vi "Qrcode Exercise Array Timeout Scan Run.vi"() -> ()   [LabVIEW 2019]
uses:
  <vilib>/userDefined/High Color/IMAQdx.ctl
  <vilib>/vision/driver/NI_Vision_Acquisition_Software.lvlib
  <vilib>/vision/NI_Vision_Development_Module.lvlib
panel:
  out "Base 3 El 3":string
  out "Base 3 El 2":string
  out "Base 3 El 1":string
  out "Base 2 El 3":string
  out "Base 2 El 2":string
  out "Base 2 El 1":string
  out "Base 1 El 3":string
  out "Base 1 El 2":string
  out "Base 1 El 1":string
  out "Base 3":string[](array[string])
  out "Base 2":string[](array[string])
  out "Base 1":string[](array[string])
  out "Index ke":i32
  out "Found?":bool
  out "Data":string
  out "Image":T1(plugin-control)
  out "Code":string
  out "Option 2":enum16{"scan", "run", "timeout"}(ring)
  out "Option":enum16{"qrcode", "lampu"}(ring)
  out "Blue":bool
  out "Green":bool
  out "Yellow":bool
  in  "Main":T2(array[cluster])=[{"Option"=enum."qrcode", "Option 2"=enum."scan", "Code"=""}, {"Option"=enum."qrcode", "Option 2"=enum."scan", "Code"=""}, {"Option"=enum."qrcode", "Option 2"=enum."scan", "Code"=""}, {"Option"=enum."qrcode", "Option 2"=enum."run", "Code"=""}, {"Option"=enum."qrcode", "Option 2"=enum."run", "Code"=""}, {"Option"=enum."qrcode", "Option 2"=enum."run", "Code"=""}, {"Option"=enum."lampu", "Option 2"=enum."timeout", "Code"=""}, {"Option"=enum."lampu", "Option 2"=enum."timeout", "Code"=""}, {"Option"=enum."lampu", "Option 2"=enum."timeout", "Code"=""}]
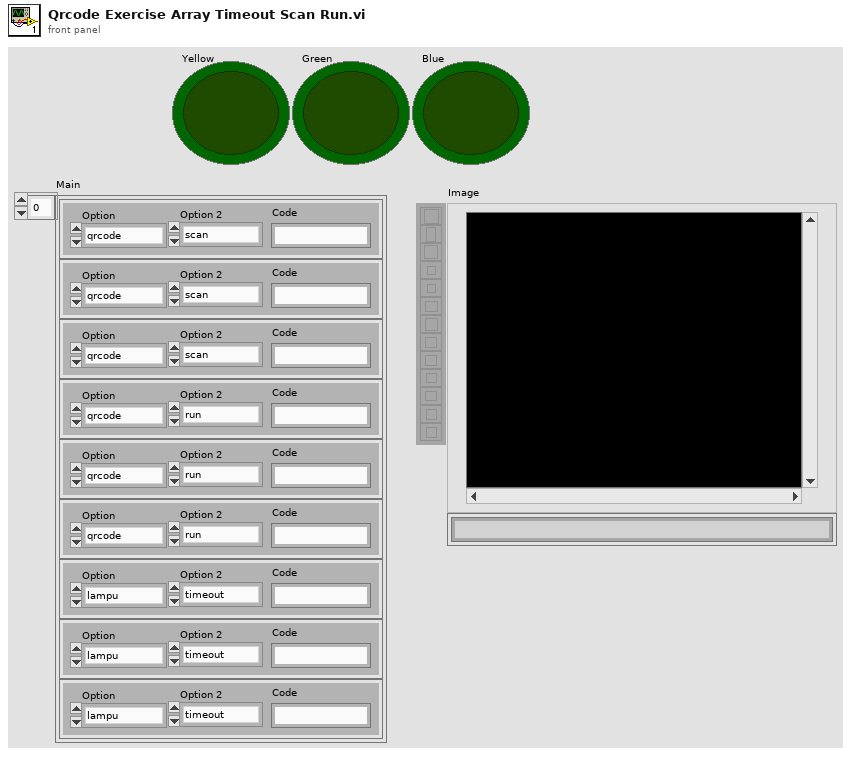
[diagram p1: front panel]
types:
  T1 = typedef "IMAQ Image.ctl" = refnum<image>
  T2 = cluster{"Option":enum16{"qrcode", "lampu"}, "Option 2":enum16{"scan", "run", "timeout"}, "Code":string}[]
  T3 = cluster{"Option":enum16{"qrcode", "lampu"}, "Option 2":enum16{"scan", "run", "timeout"}, "Code":string}
  T4 = typedef "IMAQdx.ctl" = refnum<k21>
  T5 = typedef "Image Type" = u32
  T6 = typedef "QR Code Report.ctl" = cluster{"Found?":bool, "Data":string, "Bounding Box":cluster{"x":sgl, "y":sgl}[], "Errors Corrected":u32, "Dimensions (Rows/Cols)":u32, "Version":u32, "QR Model":T7, "Stream Mode":T8, "Barcode Polarity":T9, "Mirrored?":bool, "Append Stream Position":u32, "Size of Append Stream":u32, "First EAN-128 ID":i32, "First Alternate Language ID":i32, "Append Stream ID":u32, "Minimum Edge Strength":u32, "Demodulation Mode":T10, "Cell Sample Size":T11, "Cell Filter Mode":T12}
  T7 = typedef "QR Code Model Type.ctl" = i32
  T8 = typedef "QR Code Stream Mode Type.ctl" = i32
  T9 = typedef "Data Matrix Polarity.ctl" = i32
  T10 = typedef "Demodulation Mode.ctl" = i32
  T11 = typedef "Cell Sample Size.ctl" = i32
  T12 = typedef "Cell Filter Mode.ctl" = i32
  T13 = cluster{"Option":enum16{"qrcode", "lampu"}, "Option 2":enum16{"scan", "run", "timeout"}, "Data":string}
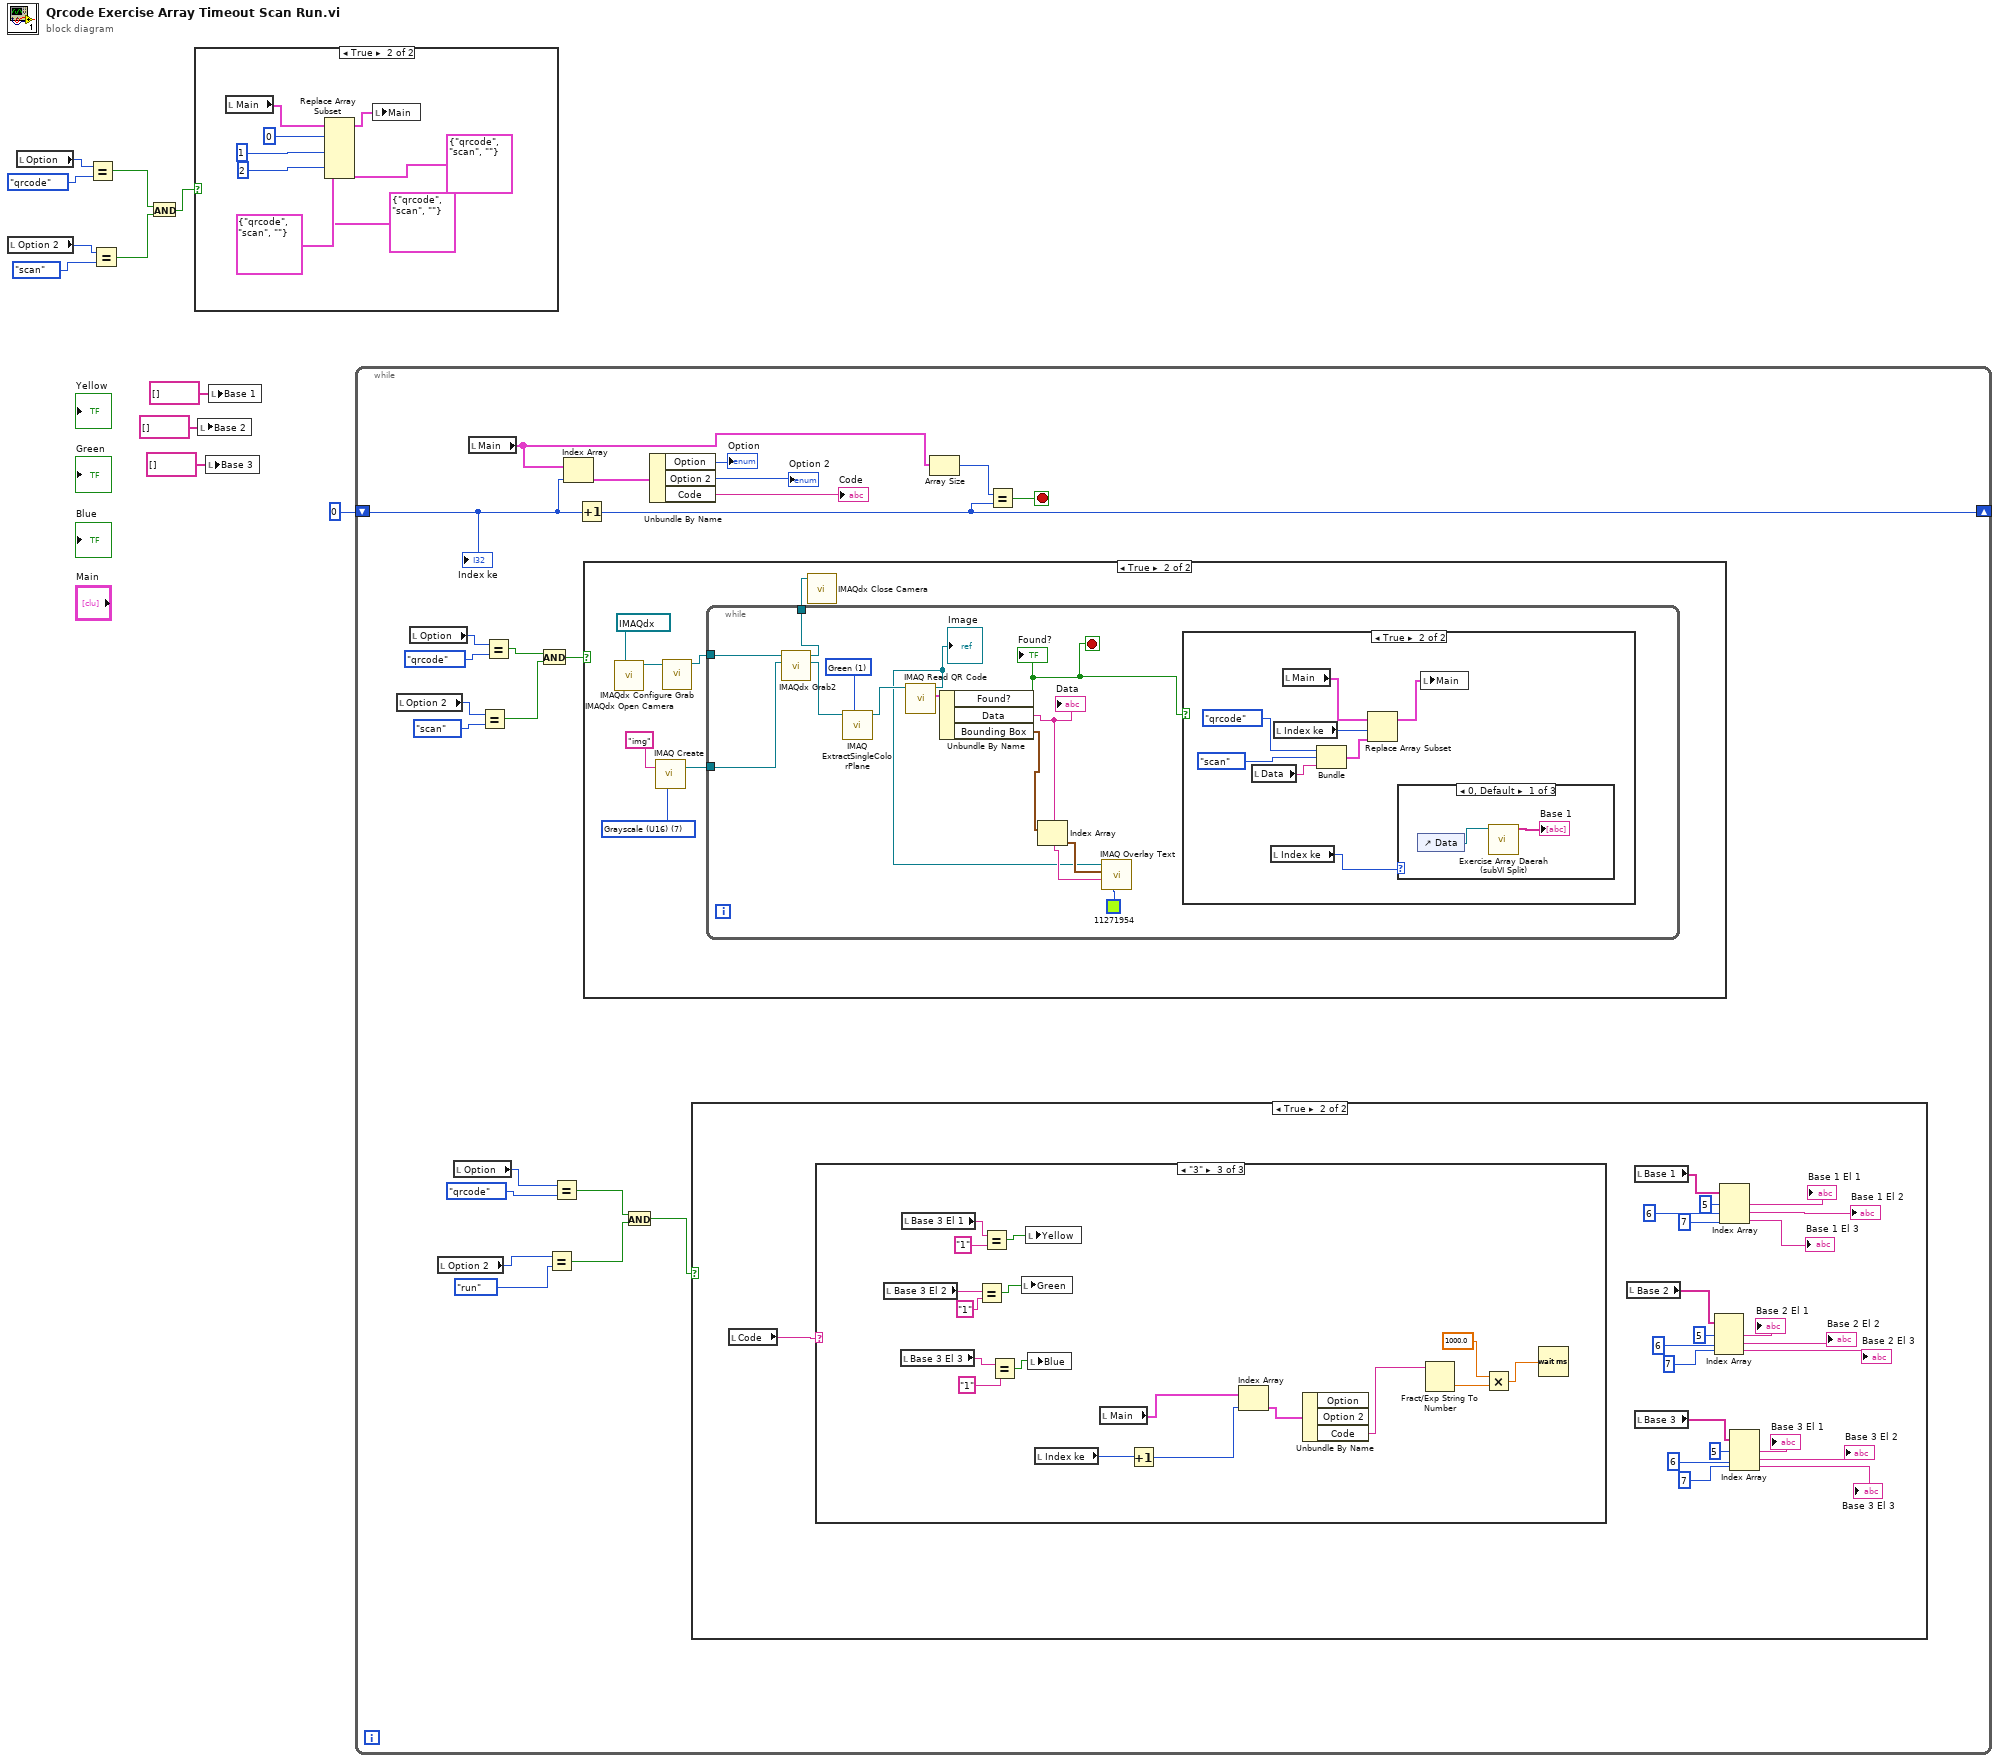
[diagram p0: block diagram]
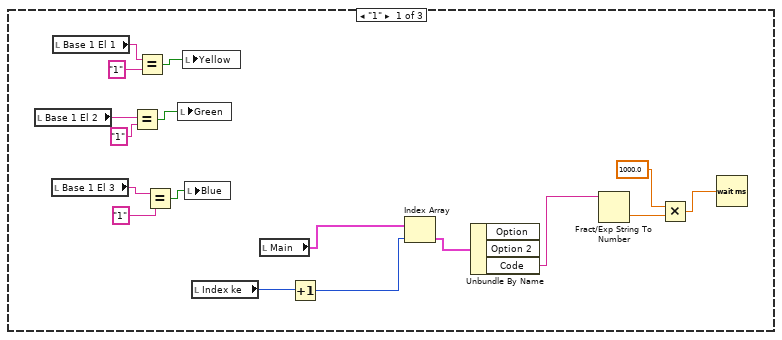
[diagram p4: hidden frame]
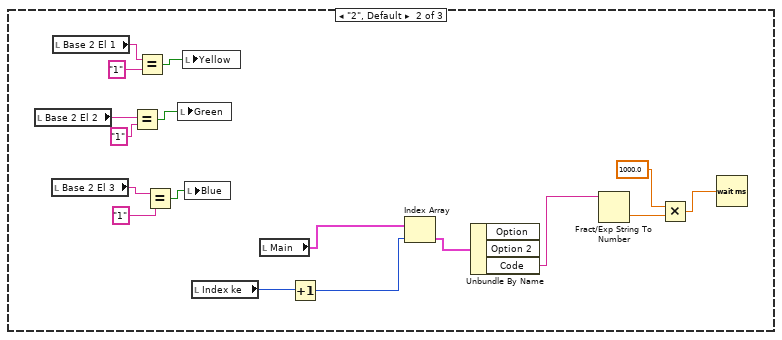
[diagram p5: hidden frame]
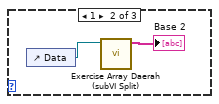
[diagram p8: hidden frame]
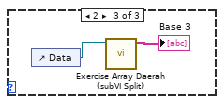
[diagram p9: hidden frame]
diagram:
  n1 = local read "Option 2"() -> (w10:enum16{"scan", "run", "timeout"})
  n2 = local read "Option"() -> (w8:enum16{"qrcode", "lampu"})
  n3 = Equal?(x=w8, y=enum16{"qrcode", "lampu"}."qrcode" ("Option")) -> (x = y?=w6:bool)
  n4 = Equal?(x=w10, y=enum16{"scan", "run", "timeout"}."scan" ("Option 2")) -> (x = y?=w5:bool)
  n5 = And(x=w6, y=w5) -> (x .and. y?=w4:bool)
  n6 = case shown="True" w4 {
    frame False {
    }
    frame True {
      n7 = local read "Main"() -> (w19:T2)
      n8 = Replace Array Subset(array=w19, new element #1=T3 {"Option"=enum."qrcode", "Option 2"=enum."scan", "Code"=""} ("new element/subarray"), index #1=0 ("index"), new element #2=T3 {"Option"=enum."qrcode", "Option 2"=enum."scan", "Code"=""} ("new element/subarray"), index #2=1 ("index"), new element #3=T3 {"Option"=enum."qrcode", "Option 2"=enum."scan", "Code"=""} ("new element/subarray"), index #3=2 ("index")) -> (w12:T2)
      n9 = local write "Main"(w12) -> ()
    }
  }
  n10 = local write "Base 2"(string[] [] ("Base 2")) -> ()
  n11 = local write "Base 3"(string[] [] ("Base 3")) -> ()
  n12 = local write "Base 1"(string[] [] ("Base 1")) -> ()
  n13 = while {
    shift-right: [w35] -> _
    shift-left: 0 -> [w42]
    stop <- w34 stop-if-true
    n14 = local read "Option 2"() -> (w32:enum16{"scan", "run", "timeout"})
    n15 = local read "Option"() -> (w31:enum16{"qrcode", "lampu"})
    n16 = local read "Option 2"() -> (w24:enum16{"scan", "run", "timeout"})
    n17 = local read "Option"() -> (w26:enum16{"qrcode", "lampu"})
    n18 = local read "Main"() -> (w37:T2)
    n19 = Equal?(x=w32, y=enum16{"scan", "run", "timeout"}."scan" ("Option 2")) -> (x = y?=w28:bool)
    n20 = Equal?(x=w31, y=enum16{"qrcode", "lampu"}."qrcode" ("Option")) -> (x = y?=w29:bool)
    n21 = And(x=w29, y=w28) -> (x .and. y?=w27:bool)
    n22 = Equal?(x=w24, y=enum16{"scan", "run", "timeout"}."run" ("Option 2")) -> (x = y?=w22:bool)
    n23 = Equal?(x=w26, y=enum16{"qrcode", "lampu"}."qrcode" ("Option")) -> (x = y?=w21:bool)
    n24 = Index Array(array=w37, index=w42) -> (element=w41:T3)
    n25 = Increment(x=w42) -> (x+1=w35:i32)
    n26 = case shown="True" w27 {
      frame False {
      }
      frame True {
        w120 = T5 7 items=["Grayscale (U8)", "Grayscale (I16)", "Grayscale (SGL)", "Complex (CSG)", "RGB (U32)", "HSL (U32)", "RGB (U64)", "Grayscale (U16)"] ("Image Type")
        n27 = call <vilib>:"IMAQdx Open Camera.vi"("Session In"=T4 "cam0") -> ("Session Out"=w122:T4)  [unwired: 9 in, 1 out]
        n28 = call "IMAQ Create"("Image Name"="img", "Image Type"=w120) -> ("New Image"=w116:T1)  [unwired: 3 in, 1 out]
        n29 = call <vilib>:"IMAQdx Configure Grab.vi"("Session In"=w122) -> ("Session Out"=w118:T4)  [unwired: 9 in, 1 out]
        n30 = while {
          tunnel: w118 -> [w135]
          tunnel: [w134] -> w117
          tunnel: w116 -> [w129]
          stop <- w123 stop-if-true
          w132 = 1 items=["Red", "Green", "Blue", "Hue", "Saturation", "Luminance", "Value", "Intensity"] ("Color Plane")
          n31 = call <vilib>:"IMAQdx Grab2.vi"("Image In"=w129, "Session In"=w135) -> ("Image Out"=w133:T1, "Session Out"=w134:T4)  [unwired: 6 in, 2 out]
          n32 = call "IMAQ ExtractSingleColorPlane"("Color Plane"=w132, "Image Src"=w133) -> ("Image Dst Out"=w131:T1)  [unwired: 8 in, 1 out]
          n33 = call "IMAQ Read QR Code"("Image"=w131) -> ("QR Code Report"=w130:T6, "Image (duplicate)"=w124:T1)  [unwired: 7 in, 2 out]
          "Image" <- w124
          n34 = Unbundle By Name(w130) -> ("Found?"=w123:bool, "Data"=w125:string, "Bounding Box"=w127:cluster{"x":sgl, "y":sgl}[])
          "Data" <- w125
          "Found?" <- w123
          n35 = Index Array(array=w127) -> (element=w126:cluster{"x":sgl, "y":sgl})  [unwired: 1 in]
          n36 = call "IMAQ Overlay Text"("Text Color (black)"=u32 11271954, "String"=w125, "Origin"=w126, "Image"=w124) -> ()  [unwired: 6 in, 2 out]
          n37 = case shown="True" w123 {
            frame False {
            }
            frame True {
              n38 = local read "Data"() -> (w139:string)
              n39 = local read "Index ke"() -> (w136:i32)
              n40 = local read "Index ke"() -> (w137:i32)
              n41 = local read "Main"() -> (w138:T2)
              n42 = Bundle("Option"=enum16{"qrcode", "lampu"}."qrcode", "Option 2"=enum16{"scan", "run", "timeout"}."scan", "Data"=w139) -> (w141:T13)  [unwired: 1 in]
              n43 = Replace Array Subset(array=w138, new element=w141, index=w137) -> (w140:T2)
              n44 = case shown="0, Default" w136 {
                frame 0, Default {
                  n45 = control-ref of="Data"() -> (w144:refnum<vi>)
                  n46 = call "Exercise Array Daerah (subVI Split).vi"("String in"=w144) -> ("Array"=→"Base 1":string[])  [unwired: 10 in]
                }
                frame 1 {
                  n47 = control-ref of="Data"() -> (w146:refnum<vi>)
                  n48 = call "Exercise Array Daerah (subVI Split).vi"("String in"=w146) -> ("Array"=→"Base 2":string[])  [unwired: 10 in]
                }
                frame 2 {
                  n49 = control-ref of="Data"() -> (w148:refnum<vi>)
                  n50 = call "Exercise Array Daerah (subVI Split).vi"("String in"=w148) -> ("Array"=→"Base 3":string[])  [unwired: 10 in]
                }
              }
              n51 = local write "Main"(w140) -> ()
            }
          }
        }
        n52 = call <vilib>:"IMAQdx Close Camera.vi"("Session In"=w117) -> ()  [unwired: 10 in, 1 out]
      }
    }
    n53 = And(x=w21, y=w22) -> (x .and. y?=w20:bool)
    n54 = Unbundle By Name(w41) -> ("Option"=→"Option":enum16{"qrcode", "lampu"}, "Option 2"=→"Option 2":enum16{"scan", "run", "timeout"}, "Code"=→"Code":string)
    n55 = case shown="True" w20 {
      frame False {
      }
      frame True {
        n56 = local read "Code"() -> (w64:string)
        n57 = case shown="\"3\"" w64 {
          frame "1" {
            n58 = local read "Base 1 El 2"() -> (w79:string)
            n59 = local read "Base 1 El 3"() -> (w80:string)
            n60 = local read "Base 1 El 1"() -> (w78:string)
            n61 = Equal?(x=w79, y="1") -> (x = y?=w73:bool)
            n62 = Equal?(x=w78, y="1") -> (x = y?=w81:bool)
            n63 = Equal?(x=w80, y="1") -> (x = y?=w74:bool)
            n64 = local write "Green"(w73) -> ()
            n65 = local write "Yellow"(w81) -> ()
            n66 = local write "Blue"(w74) -> ()
            n67 = local read "Index ke"() -> (w71:i32)
            n68 = local read "Main"() -> (w72:T2)
            n69 = Increment(x=w71) -> (x+1=w70:i32)
            n70 = Index Array(array=w72, index=w70) -> (element=w69:T3)
            n71 = Unbundle By Name(w69) -> ("Code"=w68:string)  [unwired: 2 out]
            n72 = Fract/Exp String To Number(string=w68) -> (number=w67:dbl)  [unwired: 3 in, 1 out]
            n73 = Multiply(x=1000.0, y=w67) -> (x*y=w65:dbl)
            n74 = Wait (ms)(milliseconds to wait=w65) -> ()  [unwired: 1 out]
          }
          frame "2", Default {
            n75 = local read "Base 2 El 2"() -> (w96:string)
            n76 = local read "Base 2 El 3"() -> (w97:string)
            n77 = local read "Base 2 El 1"() -> (w95:string)
            n78 = Equal?(x=w96, y="1") -> (x = y?=w90:bool)
            n79 = Equal?(x=w95, y="1") -> (x = y?=w98:bool)
            n80 = Equal?(x=w97, y="1") -> (x = y?=w91:bool)
            n81 = local write "Green"(w90) -> ()
            n82 = local write "Yellow"(w98) -> ()
            n83 = local write "Blue"(w91) -> ()
            n84 = local read "Index ke"() -> (w88:i32)
            n85 = local read "Main"() -> (w89:T2)
            n86 = Increment(x=w88) -> (x+1=w87:i32)
            n87 = Index Array(array=w89, index=w87) -> (element=w86:T3)
            n88 = Unbundle By Name(w86) -> ("Code"=w85:string)  [unwired: 2 out]
            n89 = Fract/Exp String To Number(string=w85) -> (number=w84:dbl)  [unwired: 3 in, 1 out]
            n90 = Multiply(x=1000.0, y=w84) -> (x*y=w82:dbl)
            n91 = Wait (ms)(milliseconds to wait=w82) -> ()  [unwired: 1 out]
          }
          frame "3" {
            n92 = local read "Base 3 El 2"() -> (w113:string)
            n93 = local read "Base 3 El 3"() -> (w114:string)
            n94 = local read "Base 3 El 1"() -> (w112:string)
            n95 = Equal?(x=w113, y="1") -> (x = y?=w107:bool)
            n96 = Equal?(x=w112, y="1") -> (x = y?=w115:bool)
            n97 = Equal?(x=w114, y="1") -> (x = y?=w108:bool)
            n98 = local write "Green"(w107) -> ()
            n99 = local write "Yellow"(w115) -> ()
            n100 = local write "Blue"(w108) -> ()
            n101 = local read "Index ke"() -> (w105:i32)
            n102 = local read "Main"() -> (w106:T2)
            n103 = Increment(x=w105) -> (x+1=w104:i32)
            n104 = Index Array(array=w106, index=w104) -> (element=w103:T3)
            n105 = Unbundle By Name(w103) -> ("Code"=w102:string)  [unwired: 2 out]
            n106 = Fract/Exp String To Number(string=w102) -> (number=w101:dbl)  [unwired: 3 in, 1 out]
            n107 = Multiply(x=1000.0, y=w101) -> (x*y=w99:dbl)
            n108 = Wait (ms)(milliseconds to wait=w99) -> ()  [unwired: 1 out]
          }
        }
        n109 = local read "Base 2"() -> (w53:string[])
        n110 = local read "Base 1"() -> (w63:string[])
        n111 = local read "Base 3"() -> (w52:string[])
        n112 = Index Array(array=w53, index #1=5 ("index"), index #2=6 ("index"), index #3=7 ("index")) -> (element #1=→"Base 2 El 1":string, element #2=→"Base 2 El 2":string, element #3=→"Base 2 El 3":string)
        n113 = Index Array(array=w63, index #1=5 ("index"), index #2=6 ("index"), index #3=7 ("index")) -> (element #1=→"Base 1 El 1":string, element #2=→"Base 1 El 2":string, element #3=→"Base 1 El 3":string)
        n114 = Index Array(array=w52, index #1=5 ("index"), index #2=6 ("index"), index #3=7 ("index")) -> (element #1=→"Base 3 El 1":string, element #2=→"Base 3 El 2":string, element #3=→"Base 3 El 3":string)
      }
    }
    n115 = Array Size(array=w37) -> (size(s)=w36:i32)
    n116 = Equal?(x=w36, y=w35) -> (x = y?=w34:bool)
    "Index ke" <- w42
  }
